vi "read_sub_pend_fw3.vi"(7 "instance":i32, 8 "Latest?":bool=TRUE) -> (0 "Pendulum ENC":u16, 1 "MSG CNT":u32, 2 "ENC VEL 0":u16, 3 "ENC POS 0":i32)   [LabVIEW 2022 SP3]
uses:
  LVLib/SADI_FW3.lvlib
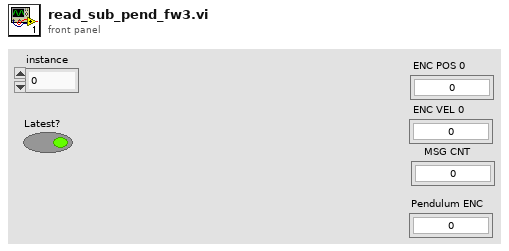
[diagram p1: front panel]
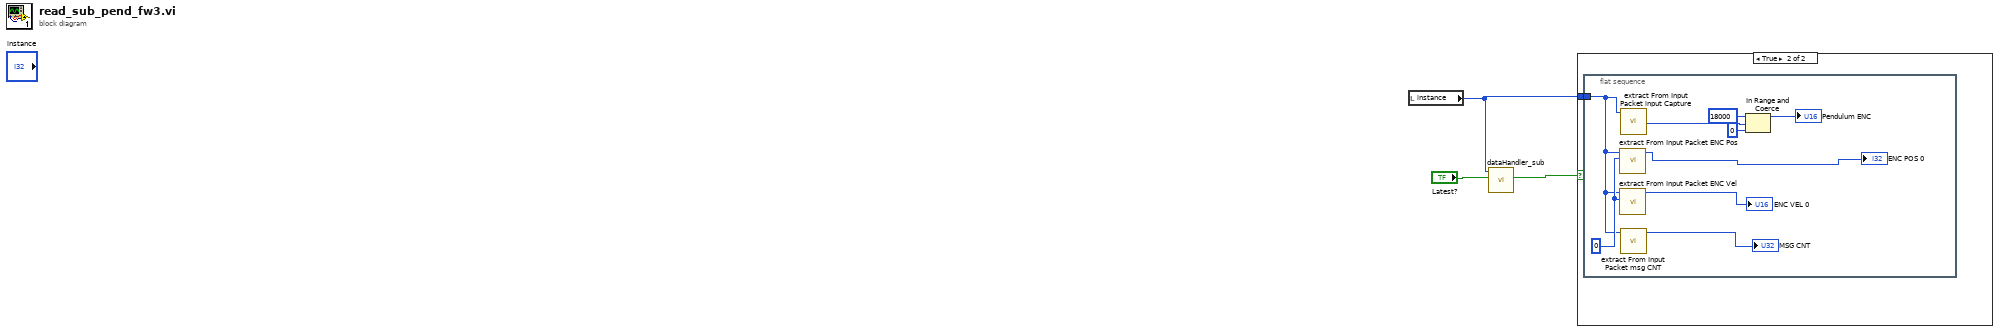
[diagram p0: block diagram]
diagram:
  n1 = local read "instance"() -> (w2:i32)
  n2 = call "dataHandler_sub.vi"("Instance"=w2, "Latest?"="Latest?") -> ("dataToRead?"=w3:bool)  [unwired: 7 in, 1 out]
  n3 = case shown="True" w3 {
    tunnel: w2 -> [_ w4]
    frame False {
    }
    frame True {
      n4 = flat-sequence {
        tunnel: w4 -> [w6]
        frame #0 {
          w13 = 0 ("channel")
          n5 = call "extract From Input Packet ENC Pos.vi"("channel"=w13, "instance"=w6) -> ("function return"=→"ENC POS 0":i32)  [unwired: 9 in]
          n6 = call "extract From Input Packet ENC Vel.vi"("channel"=w13, "instance"=w6) -> ("function return"=→"ENC VEL 0":i16)  [unwired: 9 in]
          n7 = call "extract From Input Packet input Capture.vi"("instance"=w6) -> ("function return"=w9:u16)  [unwired: 10 in]
          n8 = call "extract From Input Packet msg CNT.vi"("instance"=w6) -> ("function return"=→"MSG CNT":u32)  [unwired: 10 in]
          n9 = In Range and Coerce(upper limit=u16 18000, x=w9, lower limit=u16 0) -> (coerced(x)=→"Pendulum ENC":u16)  [unwired: 1 out]
        }
      }
    }
  }
